vi "Begin by Value.vi"(8 "Error In":errorcluster, 11 "Writer In":refnum<class "Writer.lvclass">) -> (0 "Error Out":errorcluster, 3 "Writer Out":refnum<class "Writer.lvclass">)   [LabVIEW 2017, in "LabPack.lvlib" / "Writer.lvclass"]
uses:
  Writer.lvclass
  Writer.lvclass/Writer.ctl
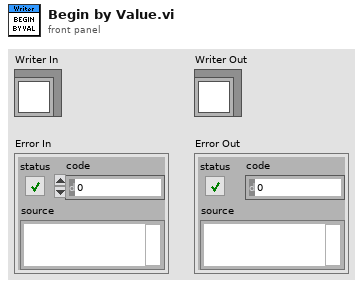
[diagram p1: front panel]
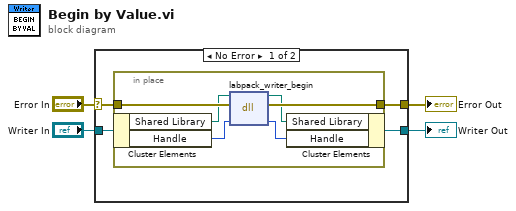
[diagram p0: block diagram]
diagram:
  n1 = case shown="No Error" "Error In" {
    selector: "Error In" -> [w8 w16]
    tunnel: [w7 w16] -> w3
    tunnel: "Writer In" -> [w6 w15]
    tunnel: [w5 w15] -> w1
    frame No Error {
      n2 = in-place {
        in-place-border: w8 -> [w14]
        in-place-border: [w13] -> w7
        n3 = in-place-cluster #1(w6) -> ("Shared Library"=w12:path, "Handle"=w10:u64)
        n4 = dll-call lib="D:/Users/cfield/Code/MessagePack/LabPack/LabVIEW/trunk/src/LabPack/Private/labpack-x64.dll" fn="labpack_writer_begin"(path in=w12, error in=w14, "writer"=w10) -> (path out=w11:path, error out=w13:errorcluster, "writer"=w9:u64)  [unwired: 2 in]
        n5 = in-place-cluster #1("Shared Library"=w11, "Handle"=w9) -> (w5:refnum<class "Writer.lvclass">)
      }
    }
    frame Error {
    }
  }
  "Error Out" <- w3
  "Writer Out" <- w1
